vi "Smart Grid.vi"(11 "EV3 in":T1) -> (3 "EV3 out":T1)   [LabVIEW 2016]
uses:
  <vilib>/NXT/Subs/LVHSConnector.ctl
  <vilib>/NXT/LegoClasses/BrickReference/BrickReference.lvclass
  <vilib>/NXT/Block Support/NXT_OutputPort.ctl
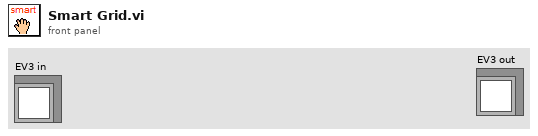
[diagram p1: front panel]
types:
  T1 = typedef "LVHSConnector.ctl" = refnum<class "BrickReference.lvclass">
  T2 = typedef "NXT_OutputPort.ctl" = u8
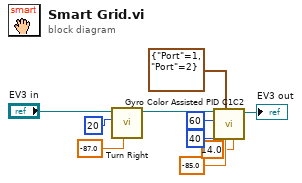
[diagram p0: block diagram]
diagram:
  n1 = call "Turn Right.vi"("Turning angle"=sgl -87.0, "Motor B (right)"=i8 20, "EV3 in"="EV3 in") -> ("EV3 out"=w7:T1)  [unwired: 8 in]
  n2 = call "Gyro Color Assisted PID C1C2.vi"("Colour 1 threshold"=sgl 14.0, "Ini. Degrees"=sgl -85.0, "Motor"=cluster{"Port":T2, "Port":T2} {"Port"=1, "Port"=2}, "De-acc"=40, "Acc"=60, "EV3 in"=w7) -> ("EV3 out"=→"EV3 out":T1)  [unwired: 5 in]
